vi "Deadband mMc.vi"(0 "deadband in":i32, 1 "Port":T1={"P type"=0, "reference"="", " Terminator "="\r\n", "Timeout"=300} {"Timeout" step=10; "P type" items=["none", "RS-232C"]}, 2 "timeout in":dbl, 3 "error in (no error)":errorcluster, 4 "set/get":bool caption="set\n\n\nget", 5 "Controller #":string) -> (6 "deadband out":i32, 7 "timeout out":dbl, 9 "error out":errorcluster)   [LabVIEW 2011]
panel:
  # "Closed loop Deadband and Timeout"
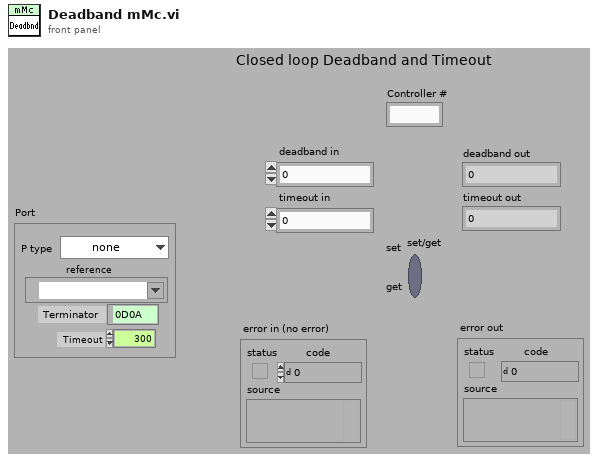
[diagram p1: front panel]
types:
  T1 = cluster{"P type":u16, "reference":refnum<visa-resource-name>, " Terminator ":string, "Timeout":i32}
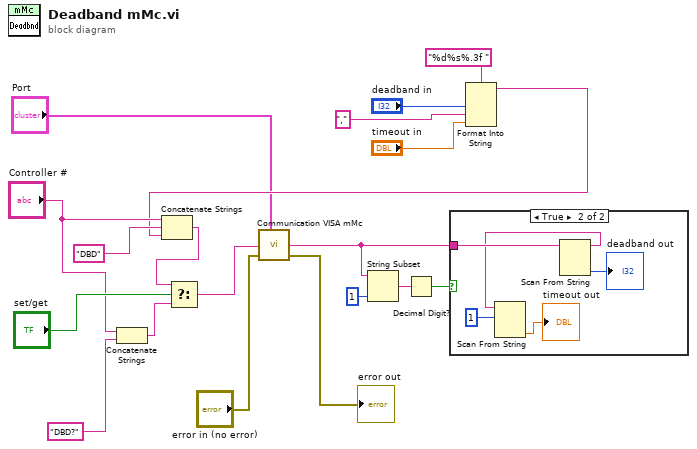
[diagram p0: block diagram]
diagram:
  n1 = Concatenate Strings("Controller #", "DBD?") -> (w19:string)
  n2 = Format Into String(format string="%d%s%.3f ", "deadband in", ",", "timeout in") -> (resulting string=w8:string)  [unwired: 2 in, 1 out]
  n3 = Concatenate Strings("Controller #", "DBD", w8) -> (w17:string)
  n4 = Select(t=w17, s="set/get", f=w19) -> (s? t:f=w16:string)
  n5 = call "Communication VISA mMc.vi"("Port"="Port", "Command"=w16, "error in (no error)"="error in (no error)") -> ("Return"=w1:string, "error out"=→"error out":errorcluster)  [unwired: 3 in, 2 out]
  n6 = String Subset(string=w1, length (rest)=1 ("length (rest)")) -> (substring=w3:string)  [unwired: 1 in]
  n7 = Decimal Digit?(1:w3) -> (0:w2:bool)
  n8 = case shown="True" w2 {
    tunnel: w1 -> [_ w23]
    frame False {
    }
    frame True {
      n9 = Scan From String(input string=w23) -> (remaining string=w22:string, output 1=→"deadband out":i32)  [unwired: 4 in, 2 out]
      n10 = Scan From String(input string=w22, initial scan location=u32 1) -> (output 1=→"timeout out":dbl)  [unwired: 3 in, 3 out]
    }
  }
